vi "Main.vi"(0 "Wait_for_Popup":bool, 5 "Run_Popup":bool, 7 "Stop":bool) -> ()   [LabVIEW 2023]
doc: "This VI is the Main VI to run the Popup VI."
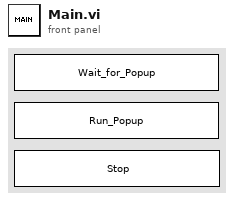
[diagram p1: front panel]
types:
  T1 = enum32{"Invalid", "Default", "Floating", "Floating/Auto-Hide", "Modal"}
  T2 = enum32{"Invalid", "Standard", "Closed", "Hidden", "Minimized", "Maximized"}
  T3 = enum32{"Bad", "Idle", "Run top level", "Running"}
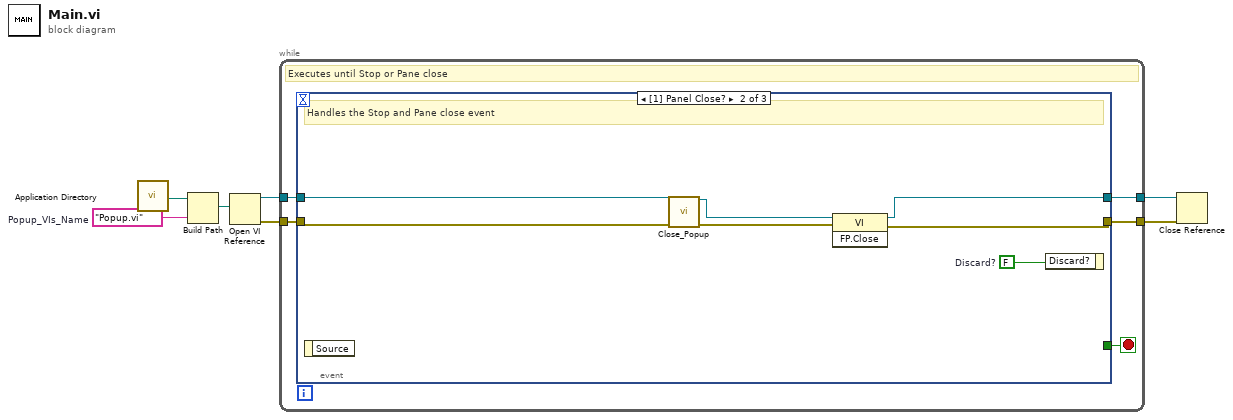
[diagram p0: block diagram]
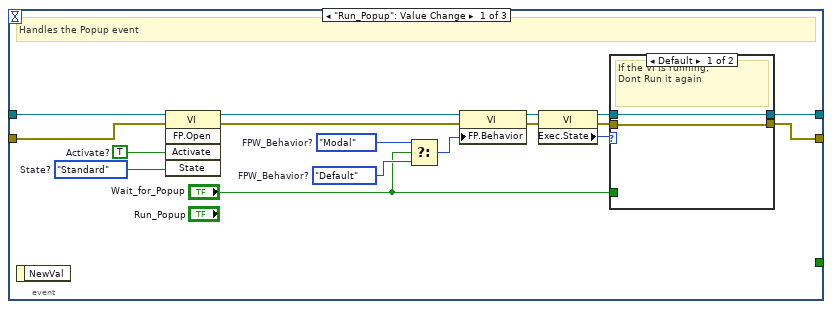
[diagram p2: hidden frame]
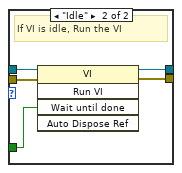
[diagram p3: hidden frame]
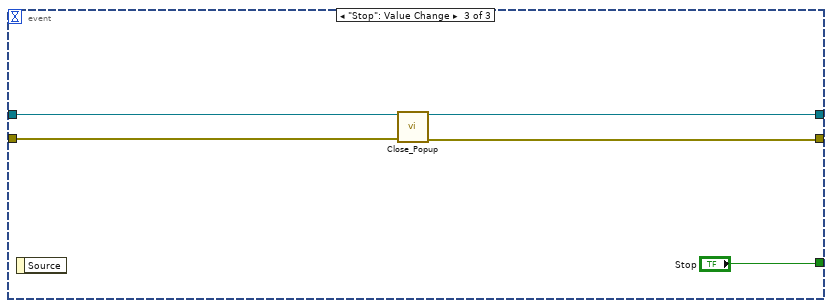
[diagram p4: hidden frame]
diagram:
  w2 = "Popup.vi"  # Popup_VIs_Name
  n1 = call <vilib>:"Application Directory.vi"() -> ("Application Directory"=w1:path)
  n2 = Build Path(base path=w1, name or relative path=w2) -> (appended path=w3:path)
  n3 = Open VI Reference(vi path=w3) -> (vi reference=w6:refnum<vi>, error out=w7:errorcluster)  [unwired: 5 in]
  n4 = while {
    tunnel: w7 -> [w11]
    tunnel: w6 -> [w10]
    tunnel: [w9] -> w5
    tunnel: [w8] -> w4
    stop <- w12 stop-if-true
    # "Executes until Stop or Pane close"
    n5 = event shown="[1] Panel Close?" {
      selector: _ -> [_ _ _]
      dyn-events: _ -> [_ _ _]
      timeout: _ -> [_ _ _]
      tunnel: [_ _ "Stop"] -> w12
      tunnel: w11 -> [w27 w37 w47]
      tunnel: w10 -> [w26 w42 w48]
      tunnel: [w14 w38 w46] -> w9
      tunnel: [w13 w40 w45] -> w8
      event "Run_Popup": Value Change {
        w22 = T1."Modal"  # FPW_Behavior?
        w23 = T1."Default"  # FPW_Behavior?
        w28 = T2."Standard"  # State?
        w29 = TRUE  # Activate?
        # "Handles the Popup event"
        n6 = event-data() -> ()  [unwired: 1 in, 1 out]
        n7 = invoke on="Invoke Node" class="VI" method="FP.Open"(reference=w26, error in=w27, "Activate"=w29, "State"=w28) -> (reference out=w25:refnum<vi>, error out=w24:errorcluster)  [unwired: 1 in, 3 out]
        n8 = Select(t=w22, s="Wait_for_Popup", f=w23) -> (s? t:f=w20:T1)
        n9 = property on="Property Node" class="VI"(reference=w25, error in=w24, "FP.Behavior"=w20) -> (reference out=w19:refnum<vi>, error out=w16:errorcluster)
        n10 = property on="Property Node" class="VI"(reference=w19, error in=w16) -> (reference out=w18:refnum<vi>, error out=w17:errorcluster, "Exec.State"=w15:T3)
        n11 = case shown="Default" w15 {
          tunnel: "Wait_for_Popup" -> [_ w36]
          tunnel: w18 -> [w31 w35]
          tunnel: w17 -> [w30 w34]
          tunnel: [w31 w33] -> w13
          tunnel: [w30 w32] -> w14
          frame Default {
            # "If the VI is running,\nDont Run it again"
          }
          frame "Idle" {
            # "If VI is idle, Run the VI"
            n12 = invoke on="Invoke Node" class="VI" method="Run VI"(reference=w35, error in=w34, "Wait until done"=w36) -> (reference out=w33:refnum<vi>, error out=w32:errorcluster)  [unwired: 2 in, 3 out]
          }
        }
      }
      event Panel Close? {
        w43 = FALSE  # Discard?
        # "Handles the Stop and Pane close event"
        n13 = event-data() -> ()  [unwired: 1 in, 1 out]
        n14 = call "Close_Popup.vi"("Reference_In"=w42, "Error_In"=w37) -> ("Reference_Out"=w41:refnum<vi>, "Error_Out"=w39:errorcluster)  [unwired: 12 in]
        n15 = invoke on="Invoke Node" class="VI" method="FP.Close"(reference=w41, error in=w39) -> (reference out=w40:refnum<vi>, error out=w38:errorcluster)  [unwired: 1 in, 1 out]
        n16 = event-data ("Event Filter Node")("Discard?"=w43) -> ()  [unwired: 1 in, 1 out]
      }
      event "Stop": Value Change {
        n17 = event-data() -> ()  [unwired: 1 in, 1 out]
        n18 = call "Close_Popup.vi"("Reference_In"=w48, "Error_In"=w47) -> ("Reference_Out"=w45:refnum<vi>, "Error_Out"=w46:errorcluster)  [unwired: 12 in]
      }
    }
  }
  n19 = Close Reference(reference=w4, error in (no error)=w5) -> ()  [unwired: 1 out]
